vi "BouncingBalls.vi"() -> ()   [LabVIEW 2021]
uses:
  <vilib>/Utility/miscctls.llb/LVBoundsTypeDef.ctl
  <vilib>/Platform/TimedLoop/XDataNode/timing_clust.ctl
  <vilib>/Platform/TimedLoop/XDataNode/nitl_modes.ctl
  <vilib>/Platform/TimedLoop/XDataNode/wakeup.ctl
  <vilib>/numeric/Random Number (Range) U64.vi
  636d1acf-31dd-47cf-9df9-c708678e367a.vi
  99d9c6ed-7766-466d-9e57-10420517a0cb.vi
  1dde9998-aa01-4f4e-9e52-5e0ab0fbb4f3.vi
  a9a4900a-2b54-4651-af54-0ae4c0897e02.vi
  30555bed-d955-4301-a4fd-91ee1136a784.vi
  daf6f0b3-705a-4ea0-a8f5-c86d5a5608bb.vi
  34f3ecef-8c6f-470c-b00b-0e50cc4f57de.vi
  <vilib>/numeric/sub_Random U32.vi
  <vilib>/platform/TimedLoop/XDataNode/XDataNode.xnode
  <vilib>/Platform/TimedLoop/XDataNode/XDNodeRunTimeDep.lvlib
panel:
  out "tEnq":u32
  out "tL5":u32
  out "tL4":u32
  out "tL3":u32
  out "tL2":u32
  out "tL1":u32
  out "nParts":i32
  out "tPhysics":i64
  out "tLoop":u32
  out "tDisp":u32
  out "tDraw":u32
  out "tDeq":u32
  out "Picture":picture
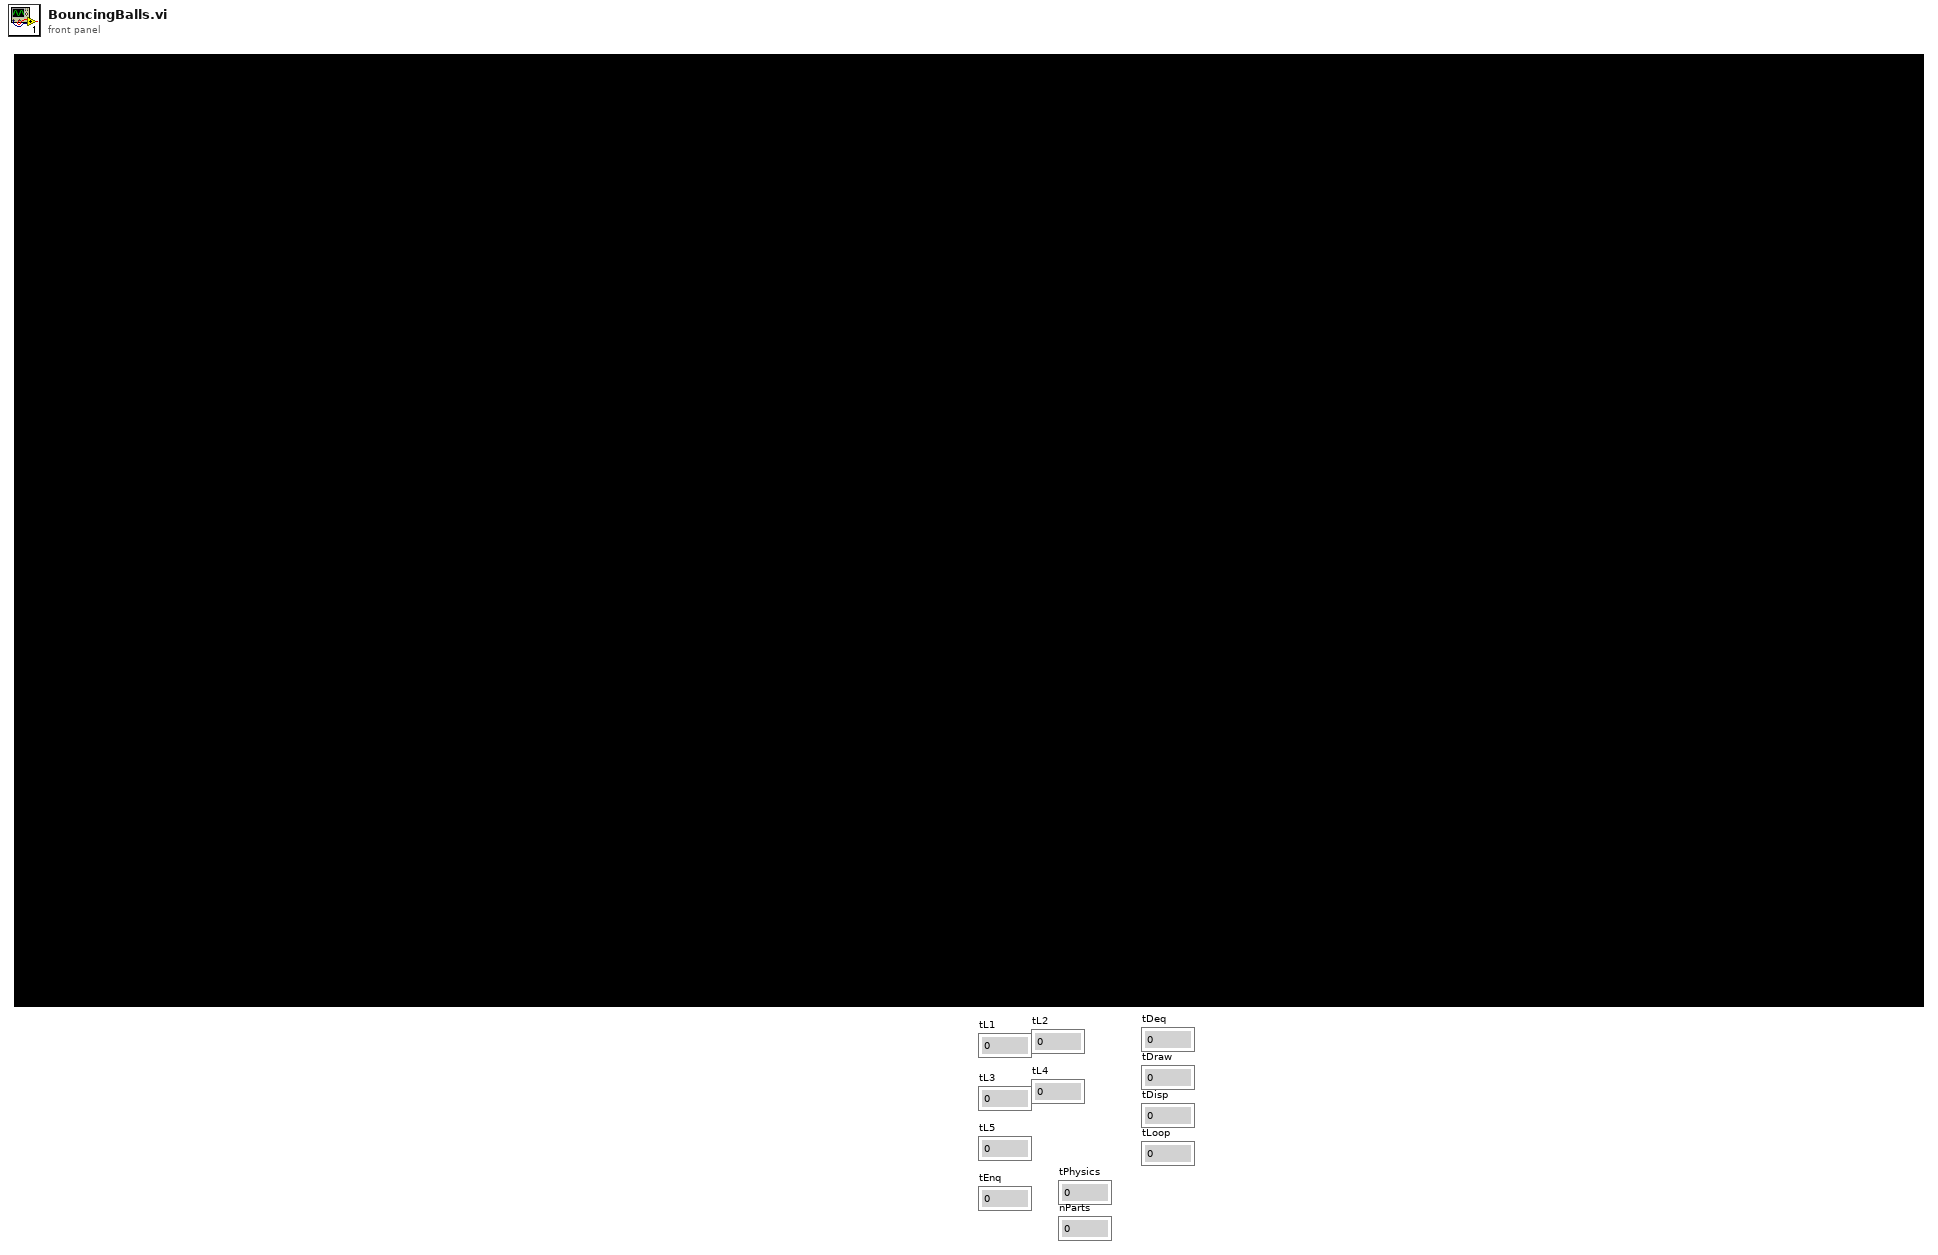
[diagram p1: front panel]
types:
  T1 = typedef "LVBoundsTypeDef.ctl" = cluster{"Width":u32, "Height":u32}
  T2 = cluster{dbl, dbl, "upper bound (100)":dbl, "upper bound (100) 2":dbl}[]
  T3 = typedef "XDNodeRunTimeDep.lvlib/timing_clust.ctl" = cluster{"Expected End [f-1]":u64, "Actual End [f-1]":u64, "Finished Late? [f-1]":bool, "Expected End [i-1]":u64, "Actual End [i-1]":u64, "Finished Late? [i-1]":bool, "Expected Start [i]":u64, "Actual Start [i]":u64, "Expected Start [f]":u64, "Actual Start [f]":u64, "Source Name":string, "Structure Name":string, "Period":i64, "Deadline":i64, "Offset":i64, "Start":i64, "Priority":i32, "Timeout":i32, "Mode":T4, "Wakeup Reason":T5, "Error":errorcluster, "Source Type":string, "Secondary Source Type":string, "Global End Time":u64, "Global Start Time":u64, "Frame Duration":u64, "Iteration Duration":u64, "Assigned CPU":i32, "I/O Scan Engine Mode":u32}
  T4 = typedef "XDNodeRunTimeDep.lvlib/nitl_modes.ctl" = enum32{"No Change", "Process missed periods, maintain original phase", "Discard missed periods, maintain original phase", "Process missed periods, ignore original phase", "Discard missed periods, ignore original phase"}
  T5 = typedef "XDNodeRunTimeDep.lvlib/wakeup.ctl" = enum32{"Normal", "Aborted", "Asynchronous wakeup", "Timing source error", "Timed loop error", "Timeout"}
  T6 = cluster{dbl, dbl, "upper bound (100)":dbl, dbl}[]
  T7 = typedef "LVPoint32TypeDef.ctl" = cluster{"Horizontal":i32, "Vertical":i32}
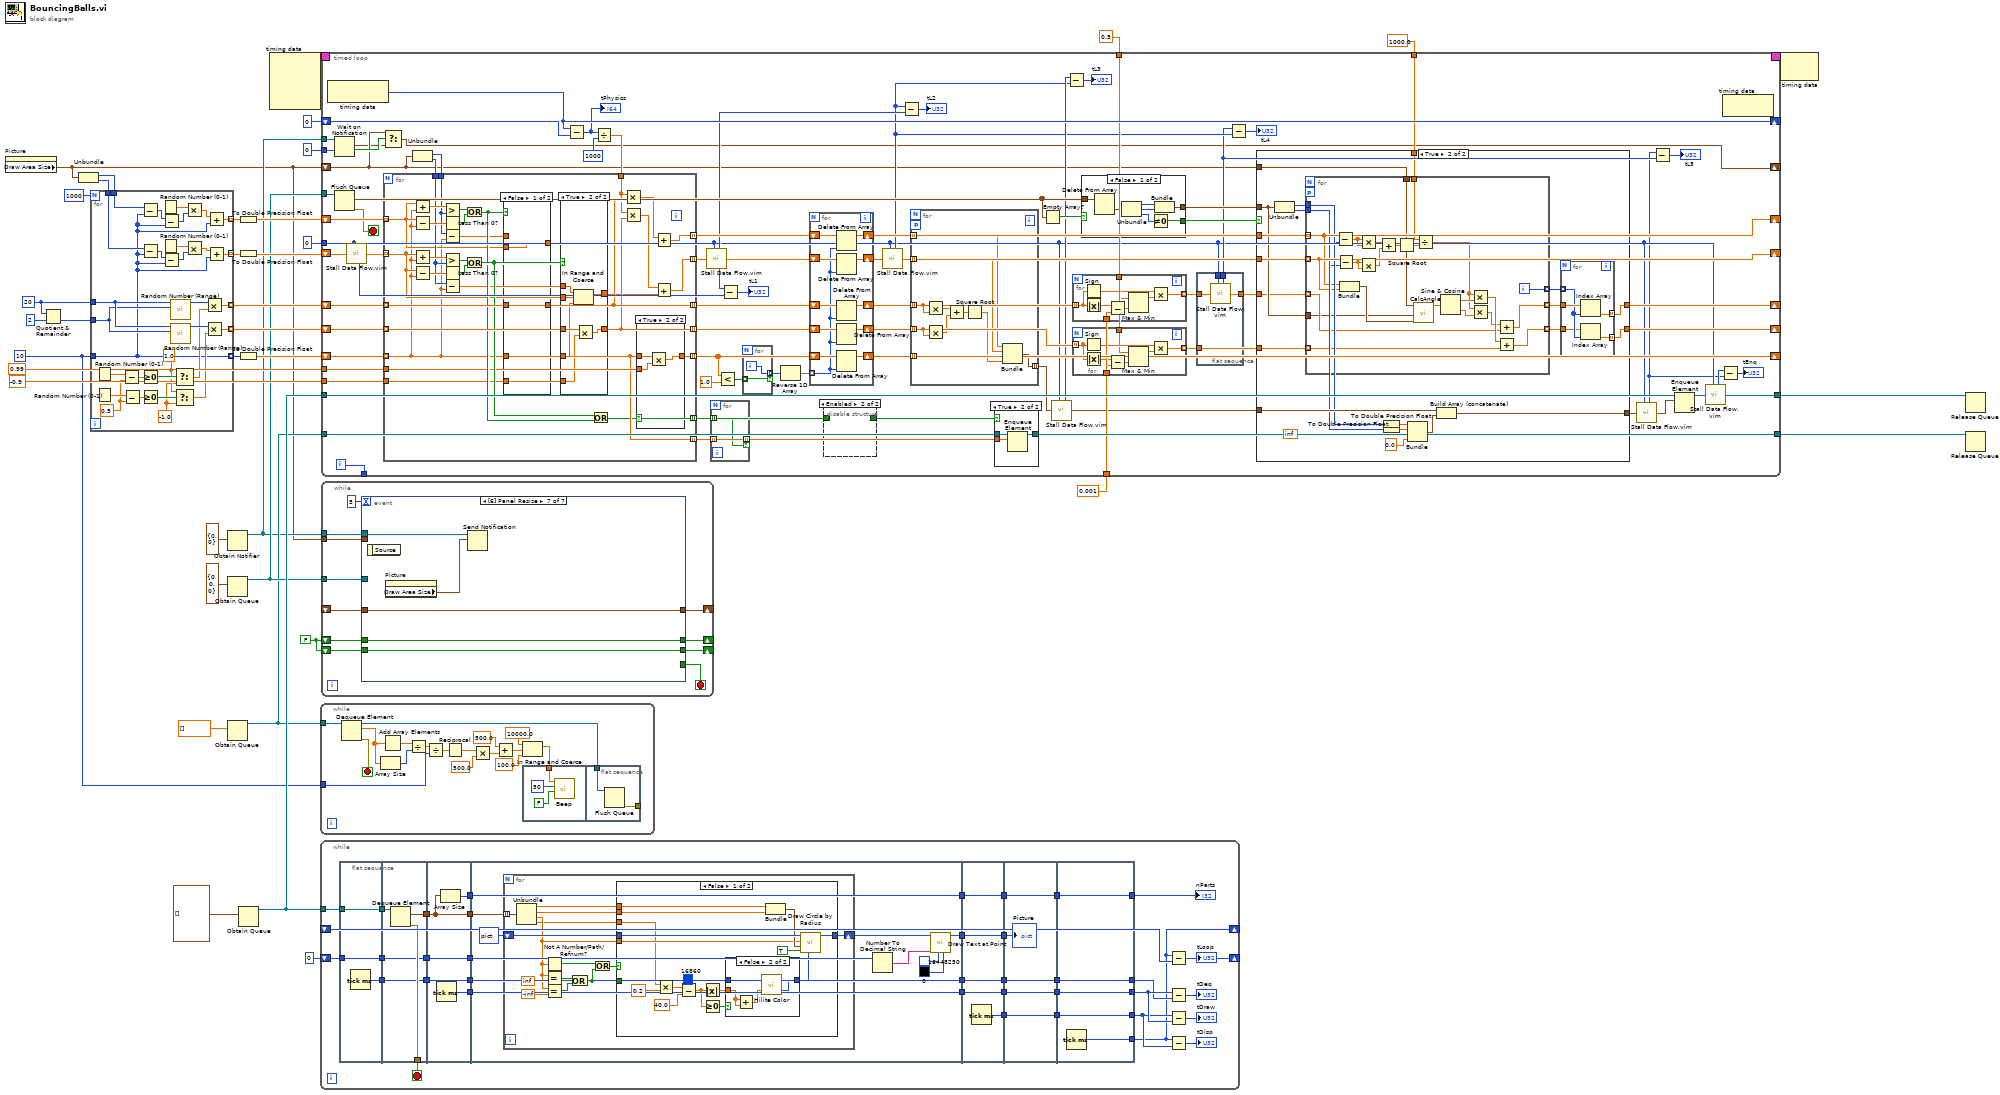
[diagram p0: block diagram]
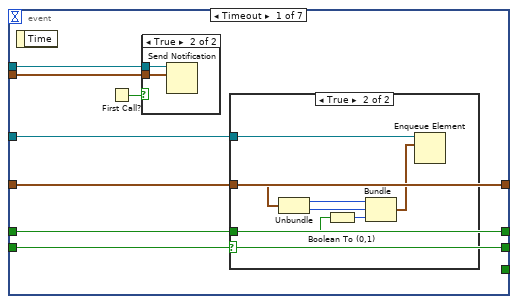
[diagram p2: hidden frame]
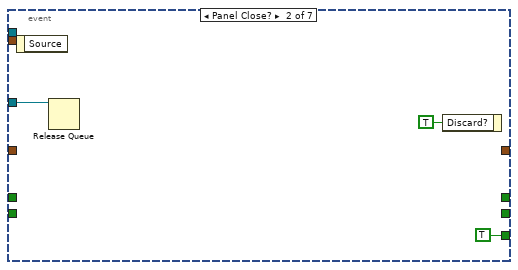
[diagram p5: hidden frame]
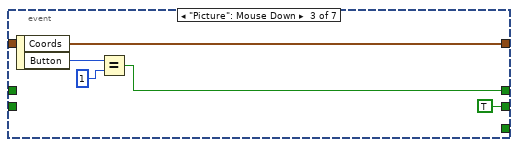
[diagram p6: hidden frame]
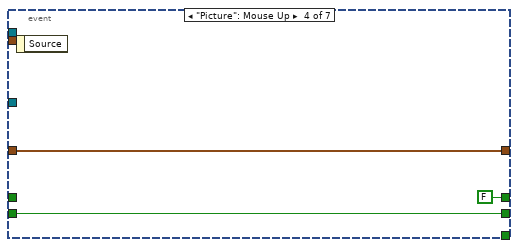
[diagram p7: hidden frame]
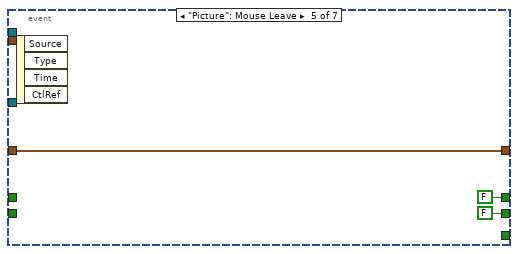
[diagram p8: hidden frame]
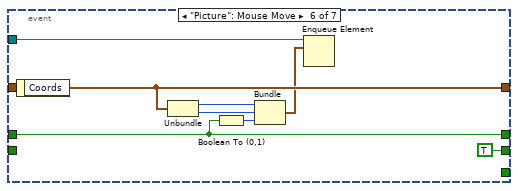
[diagram p9: hidden frame]
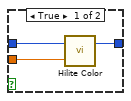
[diagram p10: hidden frame]
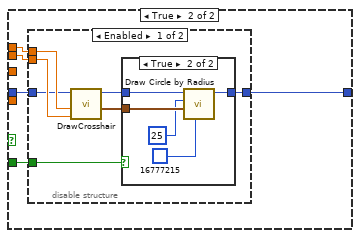
[diagram p11: hidden frame]
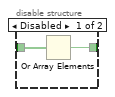
[diagram p15: hidden frame]
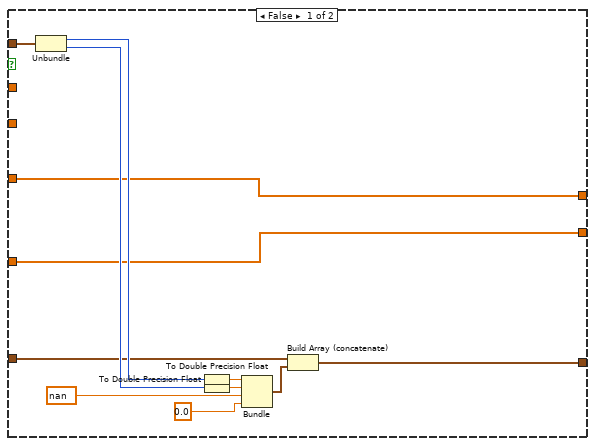
[diagram p17: hidden frame]
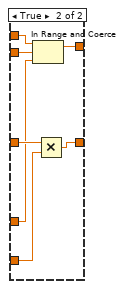
[diagram p20: hidden frame]
diagram:
  w7 = FALSE
  w9 = u64 10 ("upper bound (100)")
  w36 = u64 20 ("upper bound (100)")
  n1 = property on="Picture" class="Pict"() -> ("Draw Area Size"=w2:T1)  [unwired: 2 in, 2 out]
  n2 = Quotient & Remainder(x=w36, y=u64 2) -> (floor(x/y)=w34:u64)  [unwired: 1 out]
  n3 = Unbundle(w2) -> ("Width"=w18:u32, "Height"=w17:u32)
  n4 = for {
    N: 1000 -> [_]
    tunnel: w18 -> [w66]
    tunnel: w17 -> [w65]
    tunnel: [w42] -> w33 mode=indexing
    tunnel: [w41] -> w31 mode=indexing
    tunnel: w36 -> [w68]
    tunnel: w34 -> [w67]
    tunnel: [w59] -> w24 mode=indexing
    tunnel: [w57] -> w23 mode=indexing
    tunnel: [w39] -> w29 mode=indexing
    tunnel: w9 -> [w39]
    w51 = -1.0
    w52 = 1.0
    w62 = 0.5 ("y")
    n5 = Random Number (0-1)() -> (number: 0 to 1=w64:dbl)
    n6 = Random Number (0-1)() -> (number: 0 to 1=w63:dbl)
    n7 = Subtract(x=w64, y=w62) -> (x-y=w61:dbl)
    n8 = Subtract(x=w63, y=w62) -> (x-y=w54:dbl)
    n9 = Subtract(x=w66, y=w39) -> (x-y=w49:u64)
    n10 = Subtract(x=w65, y=w39) -> (x-y=w44:u64)
    n11 = Greater Or Equal To 0?(x=w61) -> (x >= 0?=w56:bool)
    n12 = Greater Or Equal To 0?(x=w54) -> (x >= 0?=w53:bool)
    n13 = Random Number (0-1)() -> (number: 0 to 1=w48:dbl)
    n14 = Random Number (0-1)() -> (number: 0 to 1=w45:dbl)
    n15 = Subtract(x=w49, y=w39) -> (x-y=w47:u64)
    n16 = Subtract(x=w44, y=w39) -> (x-y=w46:u64)
    n17 = call-poly <vilib>:"Random Number (Range).vi"("lower bound (0)"=w67, "upper bound (100)"=w68) -> ("number"=w60:u64)  [unwired: 9 in]
    n18 = call-poly <vilib>:"Random Number (Range).vi"("lower bound (0)"=w67, "upper bound (100)"=w68) -> ("number"=w58:u64)  [unwired: 9 in]
    n19 = Select(t=w52, s=w56, f=w51) -> (s? t:f=w55:dbl)
    n20 = Select(t=w52, s=w53, f=w51) -> (s? t:f=w50:dbl)
    n21 = Multiply(x=w48, y=w47) -> (x*y=w43:dbl)
    n22 = Multiply(x=w45, y=w46) -> (x*y=w40:dbl)
    n23 = Multiply(x=w60, y=w55) -> (x*y=w59:dbl)
    n24 = Multiply(x=w58, y=w50) -> (x*y=w57:dbl)
    n25 = Add(x=w43, y=w39) -> (x+y=w42:dbl)
    n26 = Add(x=w40, y=w39) -> (x+y=w41:dbl)
  }
  n27 = Obtain Notifier(notification data type=T1 {"Width"=0, "Height"=0} ("Draw Area Size")) -> (notifier out=w4:refnum<notifier>)  [unwired: 3 in, 2 out]
  n28 = Obtain Queue(element data type=cluster{"Horizontal":i32, "Vertical":i32, i16} {"Horizontal"=0, "Vertical"=0, 0} ("Coords")) -> (queue out=w15:refnum<queue>)  [unwired: 4 in, 2 out]
  n29 = Obtain Queue(element data type=dbl[] []) -> (queue out=w11:refnum<queue>)  [unwired: 4 in, 2 out]
  n30 = To Double Precision Float(number=w33) -> (double precision float=w32:dbl[])
  n31 = To Double Precision Float(number=w31) -> (double precision float=w30:dbl[])
  n32 = To Double Precision Float(number=w29) -> (double precision float=w28:dbl[])
  n33 = Obtain Queue(element data type=T2 []) -> (queue out=w21:refnum<queue>)  [unwired: 4 in, 2 out]
  n34 = node-c288() -> (w38:T3)  [unwired: 4 in]
  n35 = while {
    tunnel: w11 -> [w85]
    tunnel: w9 -> [w79]
    stop <- w84 stop-if-true
    n36 = Dequeue Element(queue=w85) -> (queue out=w69:refnum<queue>, element=w83:dbl[], error out=w84:errorcluster)  [unwired: 2 in, 1 out]
    n37 = Array Size(array=w83) -> (size(s)=w82:i32)
    n38 = Add Array Elements(numeric array=w83) -> (sum=w81:dbl)
    n39 = Divide(x=w81, y=w82) -> (x/y=w80:dbl)
    n40 = Divide(x=w80, y=w79) -> (x/y=w78:dbl)
    n41 = Reciprocal(x=w78) -> (1/x=w77:dbl)
    n42 = Multiply(x=w77, y=500.0) -> (x*y=w75:dbl)
    n43 = Add(x=500.0, y=w75) -> (x+y=w73:dbl)
    n44 = In Range and Coerce(upper limit=10000.0, x=w73, lower limit=100.0) -> (coerced(x)=w70:dbl)  [unwired: 1 out]
    n45 = flat-sequence {
      tunnel: w70 -> [w86]
      tunnel: w69 -> [w90]
      tunnel: [w89] -> _
      frame #0 {
        n46 = call <vilib>:"Beep.vi"("use system alert? (T)"=FALSE, "duration (msec)"=u32 50, "frequency (Hz)"=w86) -> ()  [unwired: 9 in]
      }
      frame #1 {
        n47 = Flush Queue(queue=w90) -> (error out=w89:errorcluster)  [unwired: 1 in, 2 out]
      }
    }
  }
  n48 = while {
    tunnel: w21 -> [w125]
    shift-right: [w101] -> _
    shift-left: _ -> [w102]
    shift-right: [w95] -> _
    shift-left: u32 0 -> [w91]
    stop <- w124 stop-if-true
    n49 = flat-sequence {
      tunnel: w125 -> [w130]
      tunnel: [w130] -> w122
      tunnel: [w129] -> w119
      tunnel: [w128] -> w92
      tunnel: w91 -> [w128]
      tunnel: [w134] -> w126
      tunnel: [w133] -> w124
      tunnel: w122 -> [w135]
      tunnel: [w132] -> w120
      tunnel: w119 -> [w132]
      tunnel: [w131] -> w93
      tunnel: w92 -> [w131]
      tunnel: [w138] -> w127
      tunnel: w126 -> [w138]
      tunnel: [w140] -> w123
      tunnel: [w139] -> w121
      tunnel: w120 -> [w139]
      tunnel: [w137] -> w97
      tunnel: [w136] -> w94
      tunnel: w93 -> [w136]
      tunnel: w127 -> [w150]
      tunnel: w123 -> [w149]
      tunnel: w121 -> [w148]
      tunnel: [w145] -> w118
      tunnel: [w149] -> w117
      tunnel: [w148] -> w116
      tunnel: [w147] -> w98
      tunnel: w97 -> [w147]
      tunnel: w94 -> [w142]
      tunnel: w118 -> [w212]
      tunnel: w117 -> [w211]
      tunnel: w116 -> [w210]
      tunnel: [w212] -> w114
      tunnel: [w211] -> w113
      tunnel: [w210] -> w112
      tunnel: [w209] -> w111
      tunnel: [w208] -> w99
      tunnel: w98 -> [w208]
      tunnel: w114 -> [w214]
      tunnel: w113 -> [w217]
      tunnel: w112 -> [w216]
      tunnel: w111 -> [w215]
      tunnel: [w217] -> w110
      tunnel: [w216] -> w109
      tunnel: [w215] -> w108
      tunnel: [w213] -> w100
      tunnel: w99 -> [w213]
      tunnel: [w220] -> w107
      tunnel: [w221] -> w103
      tunnel: [w222] -> w115
      tunnel: w110 -> [w222]
      tunnel: w109 -> [w221]
      tunnel: w108 -> [w220]
      tunnel: [w219] -> w101
      tunnel: [w218] -> w96
      tunnel: w100 -> [w218]
      frame #0 {
        n50 = Tick Count (ms)() -> (millisecond timer value=w129:u32)
      }
      frame #1 {
        n51 = Dequeue Element(queue=w135) -> (element=w134:T2, error out=w133:errorcluster)  [unwired: 2 in, 2 out]
      }
      frame #2 {
        n52 = Tick Count (ms)() -> (millisecond timer value=w140:u32)
        n53 = Array Size(array=w138) -> (size(s)=w137:i32)
      }
      frame #3 {
        n54 = for {
          shift-right: [w165] -> w146
          shift-left: picture data[5B] ("new picture") -> [w164]
          tunnel: w150 -> [w163] mode=indexing
          n55 = Unbundle(w163) -> (w162:dbl, w161:dbl, "upper bound (100)"=w160:dbl, "upper bound (100) 2"=w152:dbl)
          n56 = Not A Number/Path/Refnum?(number/path/refnum=w160) -> (NaN/Path/Refnum?=w155:bool)
          n57 = Equal?(x=w160, y=inf) -> (x = y?=w157:bool)
          n58 = Equal?(x=w160, y=-inf) -> (x = y?=w156:bool)
          n59 = Compound Arithmetic op=OR(w157, w156) -> (w153:bool)
          n60 = Or(x=w155, y=w153) -> (x .or. y?=w154:bool)
          n61 = case shown="False" w154 {
            tunnel: [w180 w190] -> w165
            tunnel: w164 -> [w179 w191]
            tunnel: w162 -> [w178 w193]
            tunnel: w161 -> [w177 w192]
            tunnel: w160 -> [w175 _]
            tunnel: w153 -> [_ w189]
            tunnel: w152 -> [w171 _]
            frame False {
              n62 = Multiply(x=w171, y=0.2) -> (x*y=w170:dbl)
              n63 = Subtract(x=w170, y=40.0) -> (x-y=w167:dbl)
              n64 = Absolute Value(x=w167) -> (abs(x)=w166:dbl)
              n65 = Greater Or Equal To 0?(x=w167) -> (x >= 0?=w168:bool)
              n66 = case shown="False" w168 {
                tunnel: u32 16860 ("color(black)") -> [w184 w188]
                tunnel: [w183 w187] -> w173
                tunnel: w166 -> [w182 w185]
                frame True {
                  n67 = call <vilib>:"Hilite Color.vi"("Percentage(30)"=w182, "Color In"=w184) -> ("Hilite"=w183:u32)  [unwired: 1 out]
                }
                frame False {
                  n68 = Add(x=w185, y=w185) -> (x+y=w186:dbl)
                  n69 = call <vilib>:"Hilite Color.vi"("Percentage(30)"=w186, "Color In"=w188) -> ("Shadow"=w187:u32)  [unwired: 1 out]
                }
              }
              n70 = Bundle(w178, w177) -> (w176:cluster{dbl, dbl})  [unwired: 1 in]
              n71 = call <vilib>:"Draw Circle by Radius.vi"("color(black)"=w173, "fill?(F)"=TRUE, "pixel center"=w176, "radius"=w175, "picture"=w179) -> ("new picture"=w180:picture)  [unwired: 6 in]
            }
            frame True {
              n72 = disable-structure shown="Enabled" {
                disable-tunnel: [_ w207] -> _
                disable-tunnel: w193 -> [w200 _]
                disable-tunnel: w192 -> [w199 _]
                disable-tunnel: w191 -> [w198 w207]
                disable-tunnel: [w196 _] -> w190
                disable-tunnel: w189 -> [w195 _]
                frame Enabled {
                  n73 = call "DrawCrosshair.vi"("Y"=w199, "X"=w200, "new picture in"=w198) -> ("Center"=w194:cluster{dbl, dbl}, "new picture out"=w197:picture)  [unwired: 7 in]
                  n74 = case shown="True" w195 {
                    tunnel: [w201 w205] -> w196
                    tunnel: w197 -> [w201 w206]
                    tunnel: w194 -> [_ w204]
                    frame False {
                    }
                    frame True {
                      n75 = call <vilib>:"Draw Circle by Radius.vi"("color(black)"=u32 16777215, "pixel center"=w204, "radius"=i16 25, "picture"=w206) -> ("new picture"=w205:picture)  [unwired: 7 in]
                    }
                  }
                }
                frame Disabled {
                }
              }
            }
          }
        }
        n76 = Number To Decimal String(number=w142) -> (decimal integer string=w141:string)  [unwired: 1 in]
        n77 = call <vilib>:"Draw Text at Point.vi"("BG color(transparent)"=u32 0 ("text color(black)"), "text color(black)"=u32 16448250, "text"=w141, "picture"=w146) -> ("new picture"=w145:picture)  [unwired: 6 in, 1 out]
      }
      frame #4 {
        n78 = Tick Count (ms)() -> (millisecond timer value=w209:u32)
      }
      frame #5 {
        "Picture" <- w214
      }
      frame #6 {
        n79 = Tick Count (ms)() -> (millisecond timer value=w219:u32)
      }
    }
    n80 = Subtract(x=w101, y=w102) -> (x-y=w95:u32)
    "tLoop" <- w95
    n81 = Subtract(x=w115, y=w103) -> (x-y=→"tDeq":u32)
    n82 = Subtract(x=w107, y=w115) -> (x-y=→"tDraw":u32)
    n83 = Subtract(x=w101, y=w107) -> (x-y=→"tDisp":u32)
    "nParts" <- w96
  }
  n84 = timed-loop {
    timing: w38 -> [_]
    timing-out: [_] -> w37
    shift-right: [w276] -> _
    shift-left: w32 -> [w299]
    shift-right: [w252] -> _
    shift-left: w30 -> [w259]
    shift-right: [w286] -> _
    shift-left: w24 -> [w301]
    shift-right: [w285] -> _
    shift-left: w23 -> [w300]
    shift-right: [w273] -> _
    shift-left: w28 -> [w230]
    tunnel: -0.9 ("y") -> [w298]
    tunnel: [w295] -> _
    shift-right: [w294] -> _
    shift-left: i64 0 ("Actual Start [i]") -> [w293]
    tunnel: 0.99 ("y") -> [w291]
    tunnel: w21 -> [w271]
    tunnel: [w235] -> w20
    tunnel: 0.001 -> [w270]
    tunnel: w15 -> [w288]
    tunnel: 1000.0 -> [w284]
    tunnel: w11 -> [w282]
    tunnel: [w281] -> w10
    tunnel: 0.5 -> [w269]
    tunnel: 0 -> [w234]
    shift-right: [w223] -> _
    shift-left: w2 -> [w225]
    tunnel: w4 -> [w228]
    tunnel: 0 -> [w227]
    i -> [w295]
    stop <- w268 stop-if-true
    n85 = node-c288() -> (w294:i64)  [unwired: 1 in]
    n86 = Wait on Notification(notifier=w228, timeout in ms (-1)=w227) -> (notification=w224:T1, timed out?=w226:bool)  [unwired: 2 in, 2 out]
    n87 = Flush Queue(queue=w288) -> (remaining elements=w267:cluster{"Horizontal":i32, "Vertical":i32, i16}[], error out=w268:errorcluster)  [unwired: 1 in, 1 out]
    n88 = call "Stall Data Flow.vim"("value in"=w259, "milliseconds to wait"=w234) -> ("millisecond timer value"=w255:u32, "value out"=w258:dbl[])
    n89 = Select(t=w225, s=w226, f=w224) -> (s? t:f=w223:T1)
    n90 = Unbundle(w225) -> ("Width"=w289:u32, "Height"=w290:u32)
    n91 = Subtract(x=w294, y=w293) -> (x-y=w292:i64)
    "tPhysics" <- w292
    n92 = Divide(x=w292, y=1000) -> (x/y=w296:dbl)
    n93 = for {
      tunnel: w299 -> [w430] mode=indexing
      tunnel: w258 -> [w426] mode=indexing
      tunnel: w301 -> [w446] mode=indexing
      tunnel: w300 -> [w445] mode=indexing
      tunnel: w230 -> [w424] mode=indexing
      tunnel: w289 -> [w432]
      tunnel: w290 -> [w431]
      tunnel: w298 -> [w435]
      tunnel: [w444] -> w275 mode=indexing
      tunnel: [w442] -> w274 mode=indexing
      tunnel: w296 -> [w443]
      tunnel: [w439] -> w277 mode=indexing
      tunnel: [w438] -> w257 mode=indexing
      tunnel: [w434] -> w229 mode=indexing
      tunnel: w291 -> [w433]
      tunnel: [w423] -> w262 mode=indexing
      tunnel: [w424] -> w261 mode=indexing
      n94 = Add(x=w430, y=w424) -> (x+y=w453:dbl)
      n95 = Subtract(x=w430, y=w424) -> (x-y=w454:dbl)
      n96 = Add(x=w426, y=w424) -> (x+y=w452:dbl)
      n97 = Subtract(x=w426, y=w424) -> (x-y=w451:dbl)
      n98 = Greater?(x=w453, y=w432) -> (0:w450:bool)
      n99 = Less Than 0?(x=w454) -> (x < 0?=w449:bool)
      n100 = Subtract(x=w432, y=w424) -> (x-y=w429:dbl)
      n101 = Greater?(x=w452, y=w431) -> (0:w448:bool)
      n102 = Less Than 0?(x=w451) -> (x < 0?=w447:bool)
      n103 = Subtract(x=w431, y=w424) -> (x-y=w427:dbl)
      n104 = Or(x=w450, y=w449) -> (x .or. y?=w436:bool)
      n105 = Or(x=w448, y=w447) -> (x .or. y?=w437:bool)
      n106 = case shown="False" w436 {
        tunnel: w446 -> [w469 w476]
        tunnel: w435 -> [_ w475]
        tunnel: [w469 w474] -> w444
        tunnel: w430 -> [w468 w473]
        tunnel: w429 -> [_ w472]
        tunnel: w424 -> [_ w471]
        tunnel: [w468 w470] -> w428
        frame False {
        }
        frame True {
          n107 = In Range and Coerce(upper limit=w472, x=w473, lower limit=w471) -> (coerced(x)=w470:dbl)  [unwired: 1 out]
          n108 = Multiply(x=w476, y=w475) -> (x*y=w474:dbl)
        }
      }
      n109 = case shown="True" w437 {
        tunnel: w445 -> [w460 w467]
        tunnel: w435 -> [_ w466]
        tunnel: [w460 w465] -> w442
        tunnel: w427 -> [_ w461]
        tunnel: w426 -> [w459 w464]
        tunnel: w424 -> [_ w463]
        tunnel: [w459 w462] -> w425
        frame False {
        }
        frame True {
          n110 = In Range and Coerce(upper limit=w461, x=w464, lower limit=w463) -> (coerced(x)=w462:dbl)  [unwired: 1 out]
          n111 = Multiply(x=w467, y=w466) -> (x*y=w465:dbl)
        }
      }
      n112 = Or(x=w437, y=w436) -> (x .or. y?=w423:bool)
      n113 = Multiply(x=w443, y=w444) -> (x*y=w441:dbl)
      n114 = Multiply(x=w443, y=w442) -> (x*y=w440:dbl)
      n115 = case shown="True" w423 {
        tunnel: w424 -> [w455 w458]
        tunnel: w433 -> [_ w457]
        tunnel: [w455 w456] -> w434
        frame False {
        }
        frame True {
          n116 = Multiply(x=w458, y=w457) -> (x*y=w456:dbl)
        }
      }
      n117 = Add(x=w441, y=w428) -> (x+y=w439:dbl)
      n118 = Add(x=w440, y=w425) -> (x+y=w438:dbl)
    }
    n119 = call "Stall Data Flow.vim"("value in"=w257, "milliseconds to wait"=w234) -> ("millisecond timer value"=w251:u32, "value out"=w256:dbl[])
    n120 = for {
      tunnel: w262 -> [w306] mode=indexing
      tunnel: w261 -> [w307] mode=indexing
      tunnel: [w307] -> w260 mode=indexing if=w306
    }
    n121 = Less?(x=w229, y=1.0) -> (x < y?=w279:bool[])
    n122 = Subtract(x=w251, y=w255) -> (x-y=→"tL1":u32)
    n123 = for {
      tunnel: w279 -> [w336] mode=indexing
      tunnel: [w337] -> w278 mode=indexing if=w336
      i -> [w337]
    }
    n124 = Reverse 1D Array(array=w278) -> (reversed array=w272:i32[])
    n125 = for {
      shift-right: [w334] -> w276
      shift-left: w277 -> [w335]
      shift-right: [w332] -> w253
      shift-left: w256 -> [w333]
      shift-right: [w330] -> w264
      shift-left: w275 -> [w331]
      shift-right: [w328] -> w263
      shift-left: w274 -> [w329]
      shift-right: [w326] -> w273
      shift-left: w229 -> [w327]
      tunnel: w272 -> [w325] mode=indexing
      n126 = Delete From Array(array=w335, index=w325) -> (array with subset deleted=w334:dbl[])  [unwired: 1 in, 1 out]
      n127 = Delete From Array(array=w333, index=w325) -> (array with subset deleted=w332:dbl[])  [unwired: 1 in, 1 out]
      n128 = Delete From Array(array=w331, index=w325) -> (array with subset deleted=w330:dbl[])  [unwired: 1 in, 1 out]
      n129 = Delete From Array(array=w329, index=w325) -> (array with subset deleted=w328:dbl[])  [unwired: 1 in, 1 out]
      n130 = Delete From Array(array=w327, index=w325) -> (array with subset deleted=w326:dbl[])  [unwired: 1 in, 1 out]
    }
    n131 = disable-structure shown="Enabled" {
      disable-tunnel: w262 -> [w324 _]
      disable-tunnel: [w323 _] -> w283
      frame Disabled {
        n132 = Or Array Elements(Boolean array=w324) -> (logical OR=w323:bool)
      }
      frame Enabled {
      }
    }
    n133 = call "Stall Data Flow.vim"("value in"=w253, "milliseconds to wait"=w234) -> ("millisecond timer value"=w241:u32, "value out"=w252:dbl[])
    n134 = Subtract(x=w241, y=w251) -> (x-y=→"tL2":u32)
    n135 = for {
      tunnel: w276 -> [w422] mode=indexing
      tunnel: w252 -> [w421] mode=indexing
      tunnel: w273 -> [w420] mode=indexing
      tunnel: [w419] -> w249 mode=indexing
      tunnel: w264 -> [w418] mode=indexing
      tunnel: w263 -> [w417] mode=indexing
      workers-P: _ -> [_]
      n136 = Multiply(x=w418, y=w418) -> (x*y=w416:dbl)
      n137 = Multiply(x=w417, y=w417) -> (x*y=w415:dbl)
      n138 = Add(x=w416, y=w415) -> (x+y=w414:dbl)
      n139 = Square Root(x=w414) -> (sqrt(x)=w413:dbl)
      n140 = Bundle(w422, w421, "upper bound (100)"=w420, w413) -> (w419:cluster{dbl, dbl, "upper bound (100)":dbl, dbl})  [unwired: 1 in]
    }
    n141 = case shown="True" w283 {
      tunnel: w260 -> [_ w341]
      tunnel: w282 -> [w338 w340]
      tunnel: [w338 w339] -> w281
      frame False {
      }
      frame True {
        n142 = Enqueue Element(queue=w340, element=w341) -> (queue out=w339:refnum<queue>)  [unwired: 2 in, 2 out]
      }
    }
    n143 = Empty Array?(array=w267) -> (empty?=w266:bool)
    n144 = call "Stall Data Flow.vim"("value in"=w249, "milliseconds to wait"=w234) -> ("millisecond timer value"=w247:u32, "value out"=w244:T6)
    n145 = Subtract(x=w247, y=w241) -> (x-y=→"tL3":u32)
    n146 = for {
      tunnel: w264 -> [w412] mode=indexing
      tunnel: [w409] -> w246 mode=indexing
      tunnel: w270 -> [w406]
      tunnel: w269 -> [w405]
      n147 = Sign(1:w412) -> (0:w410:dbl)
      n148 = Absolute Value(x=w412) -> (abs(x)=w411:dbl)
      n149 = Subtract(x=w411, y=w406) -> (x-y=w408:dbl)
      n150 = Max & Min(x=w405, y=w408) -> (max(x,y)=w407:dbl)  [unwired: 1 out]
      n151 = Multiply(x=w410, y=w407) -> (x*y=w409:dbl)
    }
    n152 = for {
      tunnel: w263 -> [w322] mode=indexing
      tunnel: [w319] -> w243 mode=indexing
      tunnel: w270 -> [w316]
      tunnel: w269 -> [w315]
      n153 = Sign(1:w322) -> (0:w320:dbl)
      n154 = Absolute Value(x=w322) -> (abs(x)=w321:dbl)
      n155 = Subtract(x=w321, y=w316) -> (x-y=w318:dbl)
      n156 = Max & Min(x=w315, y=w318) -> (max(x,y)=w317:dbl)  [unwired: 1 out]
      n157 = Multiply(x=w320, y=w317) -> (x*y=w319:dbl)
    }
    n158 = case shown="False" w266 {
      tunnel: w267 -> [w314 _]
      tunnel: [w310 _] -> w287
      tunnel: [w308 _] -> w265
      frame False {
        n159 = Delete From Array(array=w314) -> (deleted portion=w311:cluster{"Horizontal":i32, "Vertical":i32, i16})  [unwired: 2 in, 1 out]
        n160 = Unbundle(w311) -> ("Horizontal"=w313:i32, "Vertical"=w312:i32, w309:i16)
        n161 = Not Equal To 0?(x=w309) -> (x != 0?=w308:bool)
        n162 = Bundle("Horizontal"=w313, "Vertical"=w312) -> (w310:cluster{"Horizontal":i32, "Vertical":i32})  [unwired: 1 in]
      }
      frame True {
      }
    }
    n163 = flat-sequence {
      tunnel: w246 -> [w305]
      tunnel: [w304] -> w245
      tunnel: w234 -> [w303]
      tunnel: w243 -> [_]
      tunnel: [w302] -> w237
      frame #0 {
        n164 = call "Stall Data Flow.vim"("value in"=w305, "milliseconds to wait"=w303) -> ("millisecond timer value"=w302:u32, "value out"=w304:dbl[])
      }
    }
    n165 = Subtract(x=w237, y=w241) -> (x-y=→"tL4":u32)
    n166 = case shown="True" w265 {
      tunnel: w287 -> [w353 w370]
      tunnel: w245 -> [w344 w369]
      tunnel: [w344 w356] -> w286
      tunnel: w276 -> [_ w374]
      tunnel: w252 -> [_ w373]
      tunnel: w243 -> [w343 w368]
      tunnel: [w343 w354] -> w285
      tunnel: w284 -> [_ w372]
      tunnel: w225 -> [_ w371]
      tunnel: w244 -> [w347 w364]
      tunnel: [w345 w362] -> w240
      frame False {
        n167 = Unbundle(w353) -> ("Horizontal"=w351:i32, "Vertical"=w349:i32)
        n168 = To Double Precision Float(number=w351) -> (double precision float=w350:dbl)
        n169 = To Double Precision Float(number=w349) -> (double precision float=w348:dbl)
        n170 = Bundle(w350, w348, nan, 0.0) -> (w346:cluster{dbl, dbl, dbl, dbl})  [unwired: 1 in]
        n171 = Build Array (concatenate)(w347, w346) -> (w345:T6)
      }
      frame True {
        n172 = Unbundle(w370) -> ("Horizontal"=w360:i32, "Vertical"=w359:i32)
        n173 = for {
          tunnel: w374 -> [w396] mode=indexing
          tunnel: w373 -> [w395] mode=indexing
          tunnel: w369 -> [w387] mode=indexing
          tunnel: w368 -> [w386] mode=indexing
          tunnel: w372 -> [w398]
          tunnel: w371 -> [w397]
          tunnel: w370 -> [w383]
          tunnel: [w385] -> w357 mode=indexing
          tunnel: [w384] -> w355 mode=indexing
          tunnel: w360 -> [w382]
          tunnel: w359 -> [w381]
          workers-P: _ -> [_]
          tunnel: [w380] -> w358 mode=indexing
          i -> [w380]
          n174 = Subtract(x=w396, y=w382) -> (x-y=w404:dbl)
          n175 = Subtract(x=w395, y=w381) -> (x-y=w403:dbl)
          n176 = Bundle(w396, w395) -> (w394:cluster{dbl, dbl})  [unwired: 1 in]
          n177 = Multiply(x=w404, y=w404) -> (x*y=w402:dbl)
          n178 = Multiply(x=w403, y=w403) -> (x*y=w401:dbl)
          n179 = Add(x=w402, y=w401) -> (x+y=w400:dbl)
          n180 = Square Root(x=w400) -> (sqrt(x)=w399:dbl)
          n181 = call "CalcAngle.vi"("XY b"=w394, "XY a"=w383, "Draw Area Size"=w397) -> ("Angle (rad)"=w393:sgl)  [unwired: 7 in, 1 out]
          n182 = Divide(x=w398, y=w399) -> (x/y=w390:dbl)
          n183 = Sine & Cosine(0:w393) -> (1:w392:sgl, 2:w391:sgl)
          n184 = Multiply(x=w390, y=w392) -> (x*y=w389:dbl)
          n185 = Multiply(x=w390, y=w391) -> (x*y=w388:dbl)
          n186 = Add(x=w388, y=w387) -> (x+y=w385:dbl)
          n187 = Add(x=w389, y=w386) -> (x+y=w384:dbl)
        }
        n188 = To Double Precision Float(number=w360) -> (double precision float=w366:dbl)
        n189 = To Double Precision Float(number=w359) -> (double precision float=w365:dbl)
        n190 = Bundle(w366, w365, inf, 0.0) -> (w363:cluster{dbl, dbl, dbl, dbl})  [unwired: 1 in]
        n191 = Build Array (concatenate)(w364, w363) -> (w362:T6)
        n192 = for {
          tunnel: w358 -> [w377] mode=indexing
          tunnel: w357 -> [w379]
          tunnel: [w378] -> w356 mode=indexing
          tunnel: w355 -> [w376]
          tunnel: [w375] -> w354 mode=indexing
          n193 = Index Array(array=w379, index=w377) -> (element=w378:dbl)
          n194 = Index Array(array=w376, index=w377) -> (element=w375:dbl)
        }
      }
    }
    n195 = call "Stall Data Flow.vim"("value in"=w240, "milliseconds to wait"=w234) -> ("millisecond timer value"=w231:u32, "value out"=w239:T6)
    n196 = Subtract(x=w231, y=w237) -> (x-y=→"tL5":u32)
    n197 = Enqueue Element(queue=w271, element=w239) -> (queue out=w236:refnum<queue>)  [unwired: 2 in, 2 out]
    n198 = call "Stall Data Flow.vim"("value in"=w236, "milliseconds to wait"=w234) -> ("millisecond timer value"=w232:u32, "value out"=w235:refnum<queue>)
    n199 = Subtract(x=w232, y=w231) -> (x-y=→"tEnq":u32)
    n200 = node-c288() -> ()  [unwired: 1 in, 1 out]
  }
  n201 = while {
    shift-right: [w490] -> _
    shift-left: w7 -> [w489]
    tunnel: w15 -> [w488]
    shift-right: [w486] -> _
    shift-left: _ -> [w484]
    shift-right: [w483] -> _
    shift-left: w7 -> [w482]
    tunnel: w4 -> [w481]
    tunnel: w2 -> [w480]
    stop <- w487 stop-if-true
    n202 = event shown="[6] Panel Resize" {
      selector: _ -> [_ _ _ _ _ _ _]
      dyn-events: _ -> [_ _ _ _ _ _ _]
      timeout: 5 -> [_ _ _ _ _ _ _]
      tunnel: [w496 _ w511 FALSE FALSE w527 w532] -> w490
      tunnel: w489 -> [w496 _ _ _ _ w527 w532]
      tunnel: w488 -> [w497 w508 _ _ _ w528 _]
      tunnel: [_ TRUE _ _ _ _ _] -> w487
      tunnel: [w495 _ w512 w516 w519 w526 w533] -> w486
      tunnel: w484 -> [w495 _ _ w516 w519 _ w533]
      tunnel: [w494 _ TRUE w515 FALSE TRUE w531] -> w483
      tunnel: w482 -> [w494 _ _ w515 _ _ w531]
      tunnel: w481 -> [w493 _ _ _ _ _ w529]
      tunnel: w480 -> [w492 _ _ _ _ _ _]
      event Timeout {
        n203 = event-data() -> ()  [unwired: 1 in, 1 out]
        n204 = First Call?() -> (First Call?: T/F=w491:bool)
        n205 = case shown="True" w491 {
          tunnel: w493 -> [_ w499]
          tunnel: w492 -> [_ w498]
          frame False {
          }
          frame True {
            n206 = Send Notification(notification=w498, notifier=w499) -> ()  [unwired: 1 in, 2 out]
          }
        }
        n207 = case shown="True" w494 {
          tunnel: w497 -> [_ w506]
          tunnel: w496 -> [_ w505]
          tunnel: w495 -> [_ w500]
          frame False {
          }
          frame True {
            n208 = Unbundle(w500) -> ("Horizontal"=w504:i32, "Vertical"=w503:i32)
            n209 = Boolean To (0,1)(Boolean=w505) -> (0, 1=w502:i16)
            n210 = Bundle("Horizontal"=w504, "Vertical"=w503, w502) -> (w501:cluster{"Horizontal":i32, "Vertical":i32, i16})  [unwired: 1 in]
            n211 = Enqueue Element(queue=w506, element=w501) -> ()  [unwired: 2 in, 3 out]
          }
        }
      }
      event Panel Close? {
        n212 = event-data() -> ()  [unwired: 1 in, 1 out]
        n213 = Release Queue(queue=w508) -> ()  [unwired: 2 in, 3 out]
        n214 = event-data("Discard?"=TRUE) -> ()  [unwired: 1 in, 1 out]
      }
      event "Picture": Mouse Down {
        n215 = event-data() -> ("Coords"=w512:T7, "Button"=w514:u16)  [unwired: 1 in]
        n216 = Equal?(x=w514, y=u16 1) -> (x = y?=w511:bool)
      }
      event "Picture": Mouse Up {
        n217 = event-data() -> ()  [unwired: 1 in, 1 out]
      }
      event "Picture": Mouse Leave {
        n218 = event-data() -> ()  [unwired: 1 in, 4 out]
      }
      event "Picture": Mouse Move {
        n219 = event-data() -> ("Coords"=w526:T7)  [unwired: 1 in]
        n220 = Unbundle(w526) -> ("Horizontal"=w525:i32, "Vertical"=w524:i32)
        n221 = Boolean To (0,1)(Boolean=w527) -> (0, 1=w523:i16)
        n222 = Bundle("Horizontal"=w525, "Vertical"=w524, w523) -> (w522:cluster{"Horizontal":i32, "Vertical":i32, i16})  [unwired: 1 in]
        n223 = Enqueue Element(queue=w528, element=w522) -> ()  [unwired: 2 in, 3 out]
      }
      event Panel Resize {
        n224 = event-data() -> ()  [unwired: 1 in, 1 out]
        n225 = property on="Picture" class="Pict"() -> ("Draw Area Size"=w530:T1)  [unwired: 2 in, 2 out]
        n226 = Send Notification(notification=w530, notifier=w529) -> ()  [unwired: 1 in, 2 out]
      }
    }
  }
  n227 = node-c288(w37) -> ()  [unwired: 1 out]
  n228 = Release Queue(queue=w20) -> ()  [unwired: 2 in, 3 out]
  n229 = Release Queue(queue=w10) -> ()  [unwired: 2 in, 3 out]
